vi "Receive Message.vi"(8 "error in (no error)":errorcluster, 9 "timeout ms (-1)":i32=-1, 11 "AF Queue Stream in":refnum<class "AF Queue Stream.lvclass">) -> (0 "error out":errorcluster, 1 "Timed out?":bool, 2 "Message":refnum<class "Message.lvclass">, 3 "AF Queue Stream out":refnum<class "AF Queue Stream.lvclass">, 4 "priority":i32)   [LabVIEW 2020, in "AF Queue Stream.lvclass"]
doc: "Override this method to specify the action the local copy of this object will perform to receive a message from its remote counterpart."
uses:
  AF Queue Stream.lvclass
  <vilib>/ActorFramework/Message Dequeuer/Message Dequeuer.lvclass
  <vilib>/ActorFramework/Message Queue/Message Queue.lvclass
  <vilib>/ActorFramework/Stop Msg/Stop Msg.lvclass
  <vilib>/ActorFramework/Message/Message.lvclass
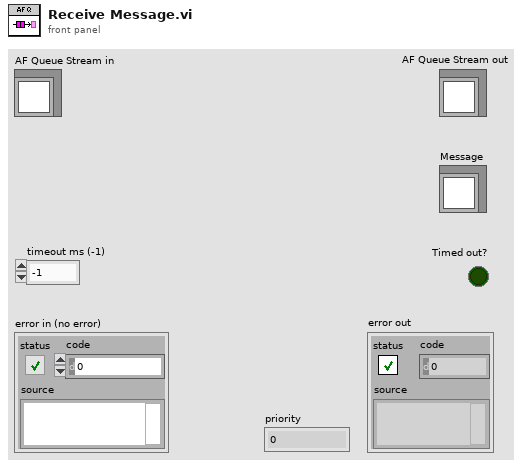
[diagram p1: front panel]
types:
  T1 = typedef "Actor Framework.lvlib/Message Dequeuer.lvclass/Dequeue Priority.ctl" = enum16{"Low", "Normal", "High", "Critical"}
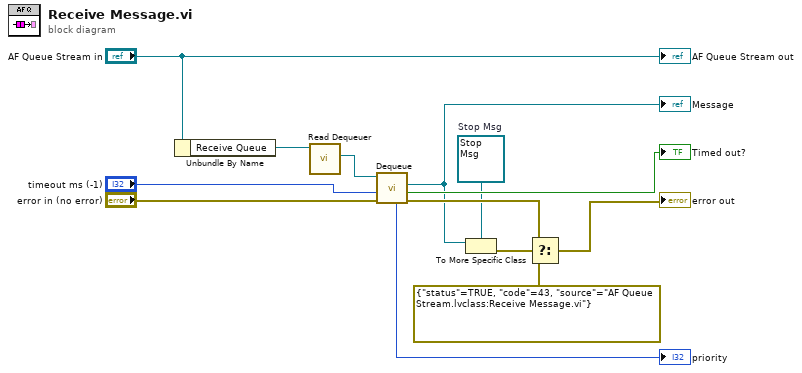
[diagram p0: block diagram]
diagram:
  w2 = refnum<class "Stop Msg.lvclass"> refnum  # Stop Msg
  n1 = Unbundle By Name("AF Queue Stream in") -> ("Receive Queue"=w8:refnum<class "Message Queue.lvclass">)
  n2 = call <vilib>:"Read Dequeuer.vi"("Message Queue"=w8) -> ("Message Dequeuer"=w7:refnum<class "Message Dequeuer.lvclass">)  [unwired: 10 in]
  n3 = call <vilib>:"Dequeue.vi"("error in (no error)"="error in (no error)", "timeout in ms (-1)"="timeout ms (-1)", "Message Dequeuer in"=w7) -> ("error out"=w6:errorcluster, "timed out?"=→"Timed out?":bool, "Message"=w3:refnum<class "Message.lvclass">, "priority"=→"priority":T1)  [unwired: 4 in, 1 out]
  "Message" <- w3
  n4 = To More Specific Class(target class=w2, reference=w3) -> (error out=w1:errorcluster)  [unwired: 1 in, 1 out]
  n5 = Select(t=w6, s=w1, f=errorcluster {"status"=TRUE, "code"=43, "source"="AF Queue Stream.lvclass:Receive Message.vi"} ("error out")) -> (s? t:f=→"error out":errorcluster)
  "AF Queue Stream out" <- "AF Queue Stream in"
